vi "Test home procedure.vi"   [LabVIEW 2011]
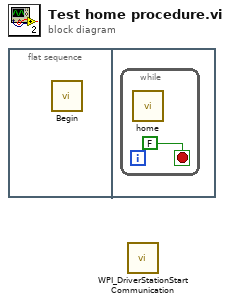
[diagram p0: block diagram]
diagram:
  n1 = flat-sequence {
    frame #0 {
      n2 = call "Begin.vi"() -> ()  [unwired: 11 in, 1 out]
    }
    frame #1 {
      n3 = while {
        stop <- FALSE stop-if-true
        n4 = call "home.vi"() -> ()  [unwired: 12 in]
      }
    }
  }
  n5 = call <vilib>:"WPI_DriverStationStart Communication.vi"() -> ()  [unwired: 12 in]
